vi "Median Filter.vi"(8 "error in (no error)":errorcluster, 10 "Database Trace":T1(array[cluster]), 11 "Database Viewer":refnum<class "Database Viewer.lvclass">) -> (0 "error out":errorcluster, 2 "Database Trace out":T1(array[cluster]), 3 "Database Viewer out":refnum<class "Database Viewer.lvclass">)   [LabVIEW 2019, in "Database Viewer.lvclass"]
uses:
  Database Viewer.lvclass
  <vilib>/Analysis/NI_AALBase.lvlib
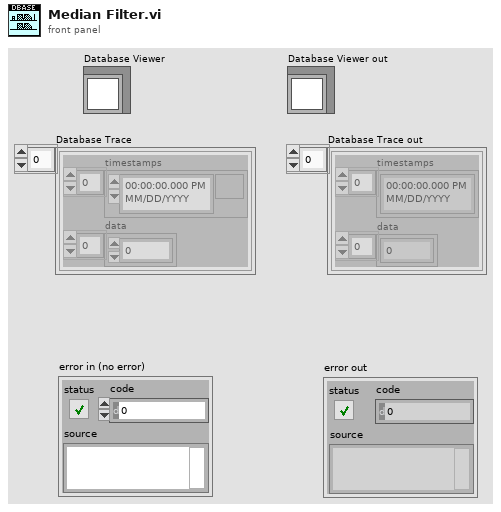
[diagram p1: front panel]
types:
  T1 = cluster{"timestamps":timestamp[], "data":dbl[]}[]
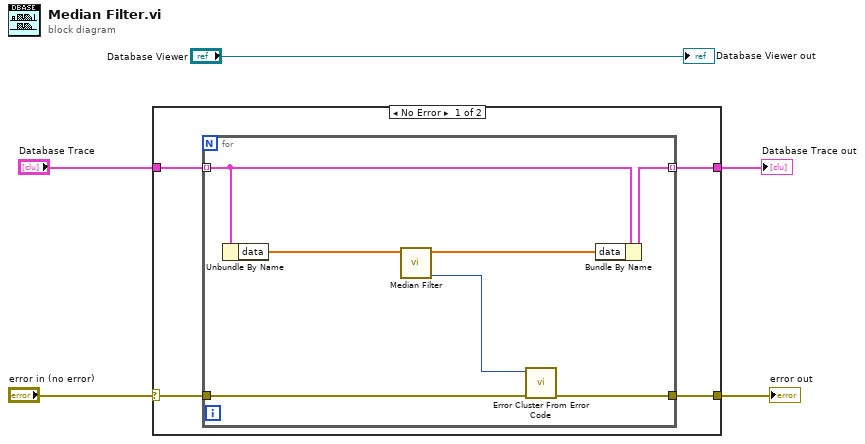
[diagram p0: block diagram]
diagram:
  n1 = case shown="No Error" "error in (no error)" {
    selector: "error in (no error)" -> [w6 w18]
    tunnel: "Database Trace" -> [w9 w17]
    tunnel: [w8 w17] -> w3
    tunnel: [w7 w18] -> w2
    frame No Error {
      n2 = for {
        tunnel: w9 -> [w16] mode=indexing
        tunnel: [w15] -> w8 mode=indexing
        tunnel: w6 -> [w11]
        tunnel: [w10] -> w7
        n3 = Unbundle By Name(w16) -> ("data"=w14:dbl[])
        n4 = call <vilib>:"Median Filter.vi"("X"=w14) -> ("error"=w12:i32, "Filtered X"=w13:dbl[])  [unwired: 9 in]
        n5 = call <vilib>:"Error Cluster From Error Code.vi"("error in (no error)"=w11, "error code (0)"=w12) -> ("error out"=w10:errorcluster)  [unwired: 7 in]
        n6 = Bundle By Name(cluster=w16, "data"=w13) -> (w15:cluster{"timestamps":timestamp[], "data":dbl[]})
      }
    }
    frame Error {
    }
  }
  "Database Trace out" <- w3
  "error out" <- w2
  "Database Viewer out" <- "Database Viewer"
